vi "DSF.Engine.Transceiver Thread.Set Debug Flags.vi"(10 "Debug Flags":refnum<class "Debug Flags.lvclass">, 11 "Transceiver Thread in":refnum<class "DSF.Engine.Transceiver Thread.lvclass">) -> (3 "Transceiver Thread out":refnum<class "DSF.Engine.Transceiver Thread.lvclass">)   [LabVIEW 2017, in "Data Sharing Framework Engine.lvlib" / "DSF.Engine.Transceiver Thread.lvclass"]
uses:
  DSF.Engine.Transceiver Thread.lvclass
  Source/Data Sharing Framework Core/Engine/Debug/Debug Flags/Debug Flags.lvclass
  DSF.Engine.Transceiver Thread.lvclass/DSF.Engine.Transceiver Thread.ctl
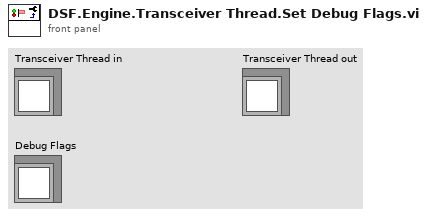
[diagram p1: front panel]
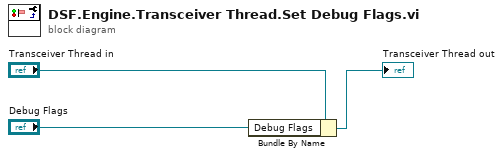
[diagram p0: block diagram]
diagram:
  n1 = Bundle By Name(cluster="Transceiver Thread in", "Debug Flags"="Debug Flags") -> (→"Transceiver Thread out":refnum<class "DSF.Engine.Transceiver Thread.lvclass">)
